vi "Select Sheet.vi"(7 "Sheet (0)":i32, 8 "error in (no error)":errorcluster, 11 "Excel Legacy in":refnum<class "Excel Legacy.lvclass">) -> (0 "error out":errorcluster, 3 "Excel Legacy out":refnum<class "Excel Legacy.lvclass">)   [LabVIEW 2013, in "Excel Legacy.lvclass"]
uses:
  Excel Legacy.lvclass
  Spreadsheet.lvclass
  Excel Legacy.lvclass/Excel Legacy.ctl
  C:/PhaeronGit/LVNPOI/Resources/NPOI 2.1.1 dotnet2/NPOI.dll
  Resources/NPOI 2.1.1 dotnet2/NPOI.dll
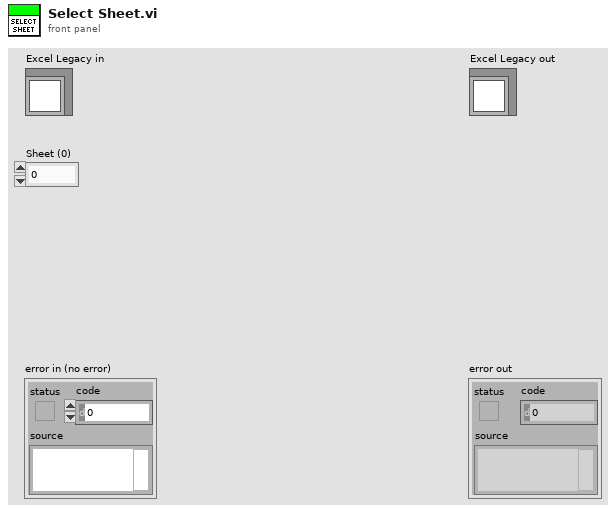
[diagram p1: front panel]
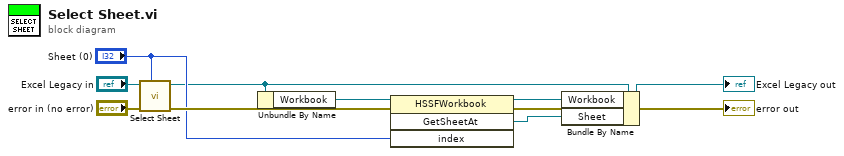
[diagram p0: block diagram]
diagram:
  n1 = call-parent "Select Sheet.vi"("Sheet (0)"="Sheet (0)", "error in (no error)"="error in (no error)", "Spreadsheet in"="Excel Legacy in") -> ("error out"=w8:errorcluster, "Spreadsheet out"=w2:refnum<class "Excel Legacy.lvclass">)  [unwired: 7 in]
  n2 = Unbundle By Name(w2) -> ("Workbook"=w1:refnum<k24>)
  n3 = invoke class="HSSFWorkbook" method="GetSheetAt"(reference=w1, error in=w8, "index"="Sheet (0)") -> (reference out=w3:refnum<k24>, error out=→"error out":errorcluster, "GetSheetAt"=w4:refnum<k24>)  [unwired: 1 in, 1 out]
  n4 = Bundle By Name(cluster=w2, "Workbook"=w3, "Sheet"=w4) -> (→"Excel Legacy out":refnum<class "Excel Legacy.lvclass">)
